vi "Compare Strings.vi"(2 "Got":string, 3 "Wanted":string) -> (0 "Reason":string, 1 "Success":bool)   [LabVIEW 2013]
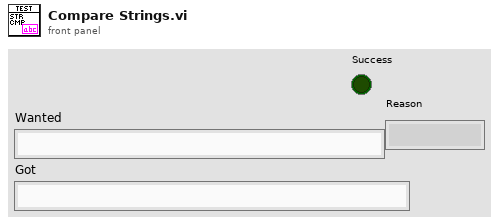
[diagram p1: front panel]
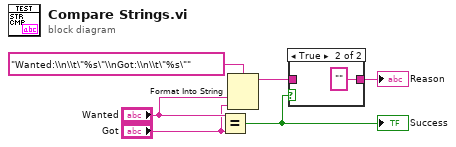
[diagram p0: block diagram]
diagram:
  n1 = Equal?(x="Wanted", y="Got") -> (x = y?=w3:bool)
  "Success" <- w3
  n2 = Format Into String(format string="Wanted:\\n\\t\"%s\"\\nGot:\\n\\t\"%s\"", "Wanted", "Got") -> (resulting string=w2:string)  [unwired: 2 in, 1 out]
  n3 = case shown="True" w3 {
    tunnel: w2 -> [w7 _]
    tunnel: [w7 ""] -> w1
    frame False {
    }
    frame True {
    }
  }
  "Reason" <- w1
